vi "Edit Config.vi"(8 "error in (no error)":errorcluster, 11 "No Out in":refnum<class "No Output.lvclass">) -> (0 "error out":errorcluster, 3 "No Out out":refnum<class "No Output.lvclass">)   [LabVIEW 2018, in "No Output.lvclass"]
doc: "No Output.lvclass:Edit Config.vi\n\nThis VI is used to edit the NI Analog configuration parameters.\n\nInstrument Communication Module Version 1.0\nOctober, 2020 Original Code Consulting Davita Bird\n www.originalcode.com"
uses:
  No Output.lvclass
  Controls/ICM Class Editor State.ctl
  Controls/ICM Editor Command.ctl
  No Output.lvclass/No Output.ctl
panel:
  in  "No Output Config":cluster{"null":dbl}
  in  "Flash Save":bool
  in  "Save":bool
  in  "Revert":bool
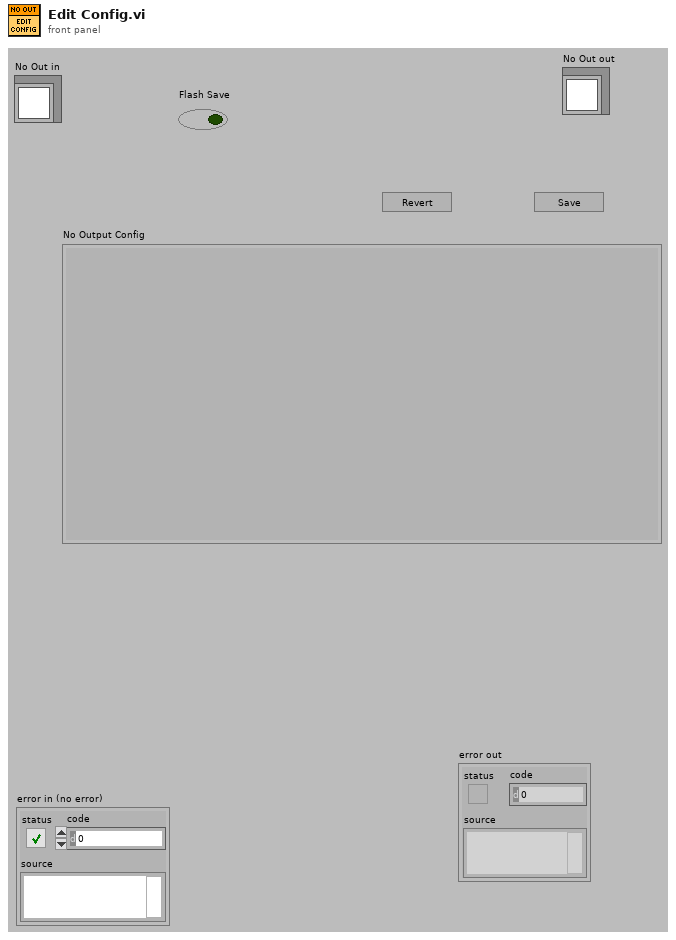
[diagram p1: front panel]
types:
  T1 = typedef "ICM Editor Command.ctl" = enum16{"No-op", "Exit"}
  T2 = typedef "ICM Class Editor State.ctl" = enum16{"Init", "Wait", "Write", "Read", "Display", "Set Flashing", "Error", "Stop"}
  T3 = typedef "Output.ctl" = cluster{"null":dbl}
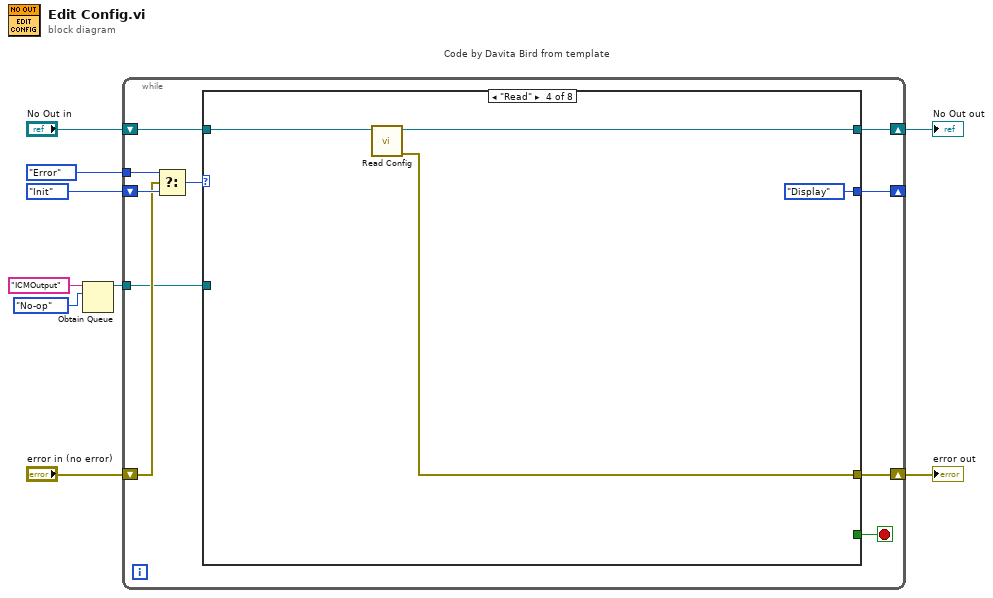
[diagram p0: block diagram]
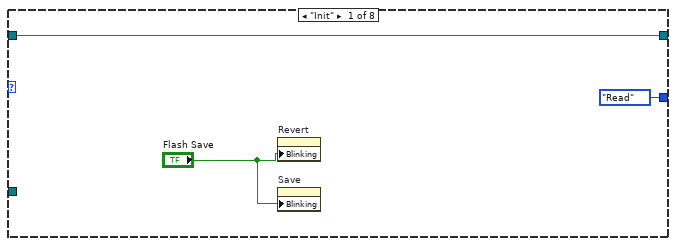
[diagram p2: hidden frame]
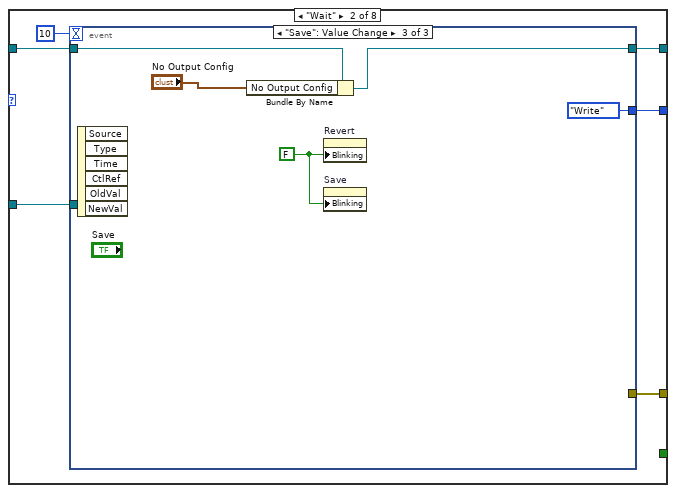
[diagram p3: hidden frame]
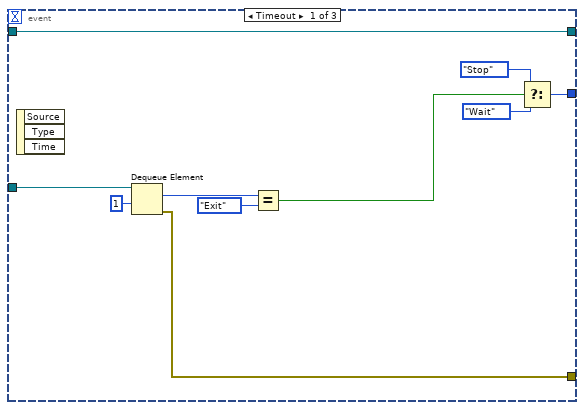
[diagram p4: hidden frame]
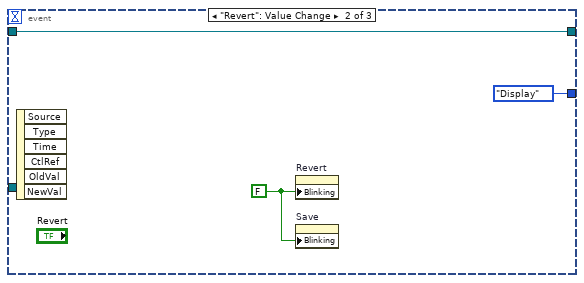
[diagram p5: hidden frame]
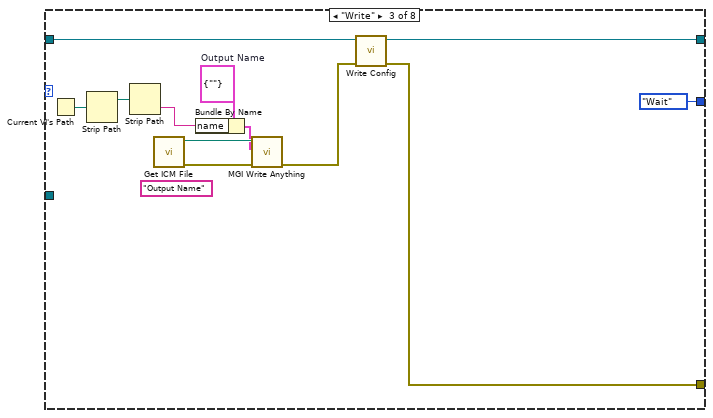
[diagram p6: hidden frame]
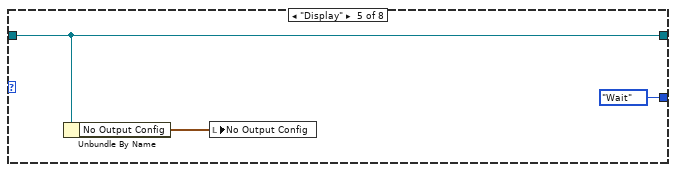
[diagram p7: hidden frame]
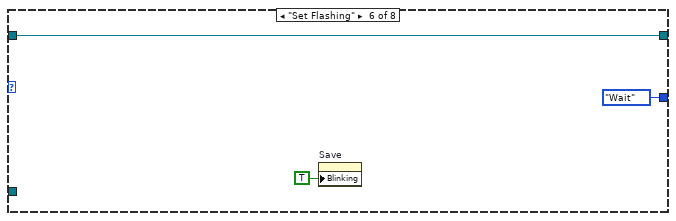
[diagram p8: hidden frame]
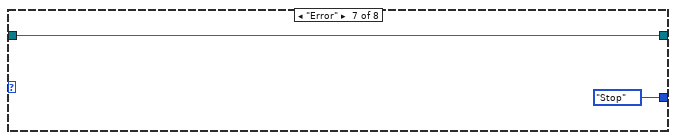
[diagram p9: hidden frame]
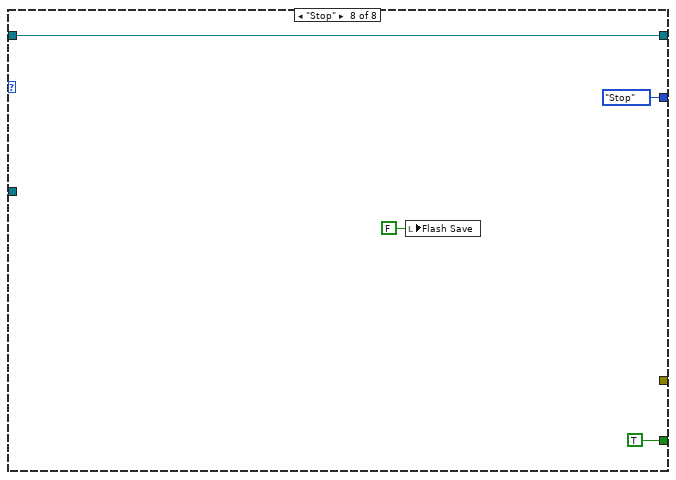
[diagram p10: hidden frame]
diagram:
  n1 = Obtain Queue(name (unnamed)="ICMOutput", element data type=ICM_Editor_Command."No-op" ("Editor Command")) -> (queue out=w1:refnum<queue>)  [unwired: 3 in, 2 out]
  n2 = while "Code by Davita Bird from template" {
    shift-right: [w19] -> w8
    shift-left: "No Out in" -> [w18]
    shift-right: [w12] -> _
    shift-left: ICM_Class_Editor_State."Init" ("Config State") -> [w16]
    shift-right: [w11] -> w6
    shift-left: "error in (no error)" -> [w14]
    tunnel: ICM_Class_Editor_State."Error" ("Config State") -> [w13]
    tunnel: w1 -> [w10]
    stop <- w17 stop-if-true
    n3 = Select(t=w13, s=w14, f=w16) -> (s? t:f=w15:T2)
    n4 = case shown="\"Read\"" w15 {
      tunnel: [w21 w26 w56 w60 w65 w68 w70 w74] -> w19
      tunnel: w18 -> [w21 w25 w57 w62 w65 w68 w70 w74]
      tunnel: [_ _ _ _ _ _ _ TRUE] -> w17
      tunnel: [ICM_Class_Editor_State."Read" ("Config State") w27 ICM_Class_Editor_State."Wait" ("Config State") ICM_Class_Editor_State."Display" ("Config State") ICM_Class_Editor_State."Wait" ("Config State") ICM_Class_Editor_State."Wait" ("Config State") ICM_Class_Editor_State."Stop" ("Config State") ICM_Class_Editor_State."Stop" ("Config State")] -> w12
      tunnel: [_ w23 w55 w61 _ _ _ _] -> w11
      tunnel: w10 -> [_ w24 _ _ _ _ _ _]
      frame "Init" {
        n5 = property on="Revert" class="Bool"("Blinking"="Flash Save") -> ()  [unwired: 2 in, 2 out]
        n6 = property on="Save" class="Bool"("Blinking"="Flash Save") -> ()  [unwired: 2 in, 2 out]
      }
      frame "Wait" {
        n7 = event shown="[2] \"Save\": Value Change" {
          selector: _ -> [_ _ _]
          dyn-events: _ -> [_ _ _]
          timeout: 10 -> [_ _ _]
          tunnel: [w35 ICM_Class_Editor_State."Display" ("Config State") ICM_Class_Editor_State."Write" ("Config State")] -> w27
          tunnel: [w38 w40 w44] -> w26
          tunnel: w25 -> [w38 w40 w45]
          tunnel: w24 -> [w37 _ _]
          tunnel: [w29 _ _] -> w23
          event Timeout {
            n8 = event-data() -> ()  [unwired: 1 in, 3 out]
            n9 = Dequeue Element(queue=w37, timeout in ms (-1)=1) -> (element=w34:T1, error out=w29:errorcluster)  [unwired: 1 in, 2 out]
            n10 = Equal?(x=w34, y=ICM_Editor_Command."Exit") -> (x = y?=w32:bool)
            n11 = Select(t=ICM_Class_Editor_State."Stop" ("Config State"), s=w32, f=ICM_Class_Editor_State."Wait" ("Config State")) -> (s? t:f=w35:T2)
          }
          event "Revert": Value Change {
            w39 = FALSE ("Blinking")
            n12 = event-data() -> ()  [unwired: 1 in, 6 out]
            n13 = property on="Revert" class="Bool"("Blinking"=w39) -> ()  [unwired: 2 in, 2 out]
            n14 = property on="Save" class="Bool"("Blinking"=w39) -> ()  [unwired: 2 in, 2 out]
          }
          event "Save": Value Change {
            w43 = FALSE ("Blinking")
            n15 = event-data() -> ()  [unwired: 1 in, 6 out]
            n16 = Bundle By Name(cluster=w45, "No Output Config"="No Output Config") -> (w44:refnum<class "No Output.lvclass">)
            n17 = property on="Revert" class="Bool"("Blinking"=w43) -> ()  [unwired: 2 in, 2 out]
            n18 = property on="Save" class="Bool"("Blinking"=w43) -> ()  [unwired: 2 in, 2 out]
          }
        }
      }
      frame "Write" {
        w49 = cluster{"name":string} {"name"=""}  # Output Name
        (unwired) "Output Name" ("Section Name (Name of \"Anything\")")
        n19 = Current VI's Path() -> (path=w54:path)
        n20 = Strip Path(path=w54) -> (stripped path=w53:path)  [unwired: 1 out]
        n21 = Strip Path(path=w53) -> (name=w48:string)  [unwired: 1 out]
        n22 = call "Get ICM File.vi"() -> ("error out"=w51:errorcluster, "ICM File"=w52:path)  [unwired: 10 in]
        n23 = Bundle By Name(cluster=w49, "name"=w48) -> (w47:cluster{"name":string})
        n24 = call <userlib>:"MGI Write Anything.vi"("Error In"=w51, "Anything"=w47, "Path (dialog)"=w52) -> ("Error Out"=w50:errorcluster)  [unwired: 6 in, 2 out]
        n25 = call-dynamic "Write Config.vi"("error in (no error)"=w50, "No Out in"=w57) -> ("error out"=w55:errorcluster, "No Out out"=w56:refnum<class "No Output.lvclass">)  [unwired: 8 in]
      }
      frame "Read" {
        n26 = call-dynamic "Read Config.vi"("No Out in"=w62) -> ("error out"=w61:errorcluster, "No Out out"=w60:refnum<class "No Output.lvclass">)  [unwired: 9 in]
      }
      frame "Display" {
        n27 = Unbundle By Name(w65) -> ("No Output Config"=w64:T3)
        n28 = local write "No Output Config"(w64) -> ()
      }
      frame "Set Flashing" {
        n29 = property on="Save" class="Bool"("Blinking"=TRUE) -> ()  [unwired: 2 in, 2 out]
      }
      frame "Error" {
      }
      frame "Stop" {
        n30 = local write "Flash Save"(FALSE ("Flash Save")) -> ()
      }
    }
  }
  "error out" <- w6
  "No Out out" <- w8
